vi "target.vi"() -> ()   [LabVIEW 2020]
uses:
  <vilib>/rvi/DataTransferAndStorage/Container/Common/niFpgaContainerGetUniqueNameForEmu.vi
  <vilib>/rvi/DataTransferAndStorage/Container/Common/niFpgaContainerSetEmuInfo.vi
  <vilib>/rvi/eio/common/nirviEmuReportErrorAndStop.vi
  <vilib>/rvi/Emulation/niFpgaGetClockAttributes.vi
  <vilib>/rvi/Emulation/niFpgaSctlEmulationGetInTimedLoop.vi
  <vilib>/rvi/Emulation/niFpgaEmulationReportErrorSimple.vi
  <vilib>/rvi/DataTransferAndStorage/Container/Common/niFpgaContainerExecOnDevCompGetState.vi
  <vilib>/rvi/Emulation/niFpgaEmulationIsFPGAContextNoSignature.vi
  <vilib>/rvi/errors/niFpgaSetErrorForExecOnDevCompSimple.vi
  <vilib>/rvi/FIFO/Fifo_Resource/nirvififoEmulationSetSize.vi
  <vilib>/rvi/FIFO/Fifo_Resource/nirviFifoEmulationQueueMgr.vi
  <instcachedir>/0/nirviFifoEmulationQueueMgr_E5CAEC123FF24DC58D834DCA3CDAA9B5.lvgen/nirviFifoEmulationQueueMgr_E5CAEC123FF24DC58D834DCA3CDAA9B5_004.vi
  <vilib>/rvi/FIFO/Fifo_Resource/nirvififoEmulationDetermineInputValidOut.vi
  <vilib>/rvi/FIFO/Fifo_Resource/nirvififoEmulationCreateLock.vi
  <vilib>/rvi/Emulation/niFpgaProcessEmulError.vi
  <vilib>/rvi/FIFO/Fifo_Resource/nirvififoEmulationObtainLock.vi
  <vilib>/rvi/FIFO/Fifo_Resource/nirvififoEmulationReleaseLock.vi
  <vilib>/rvi/occurrence/nirviWaitOnOccurrenceBase.vi
  <vilib>/rvi/errors/nirviReportUnexpectedCaseInternalError.vi
  <vilib>/rvi/errors/nirviReportUnexpectedCaseInternalError (U32).vi
  <vilib>/Utility/error.llb/Clear Errors.vi
  <vilib>/rvi/interface/RandomDataEmulation/niFpgaRandomDataHandleErrors.vi
  <vilib>/rvi/Emulation/niFpgaCriticalErrorInLSC.vi
  <vilib>/rvi/LocalResourceManager/LocalResourceManager.xnode
  <vilib>/rvi/DataTransferAndStorage/Container/XNode/niFpgaContainer.xnode
  <vilib>/rvi/FIFO/Fifo_Resource/niFpgaFifoEmulationRefIn.vi
  <vilib>/rvi/interface/RandomDataEmulation/nirviRandomDataFpgaReadWriteTemplate.vi
  <vilib>/eio/EIONode/EIONode.xnode
  <vilib>/rvi/eio/common/nirviEmuTemplateMethod_errors.vi
panel:
  out "x > y?":bool
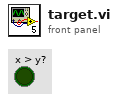
[diagram p1: front panel]
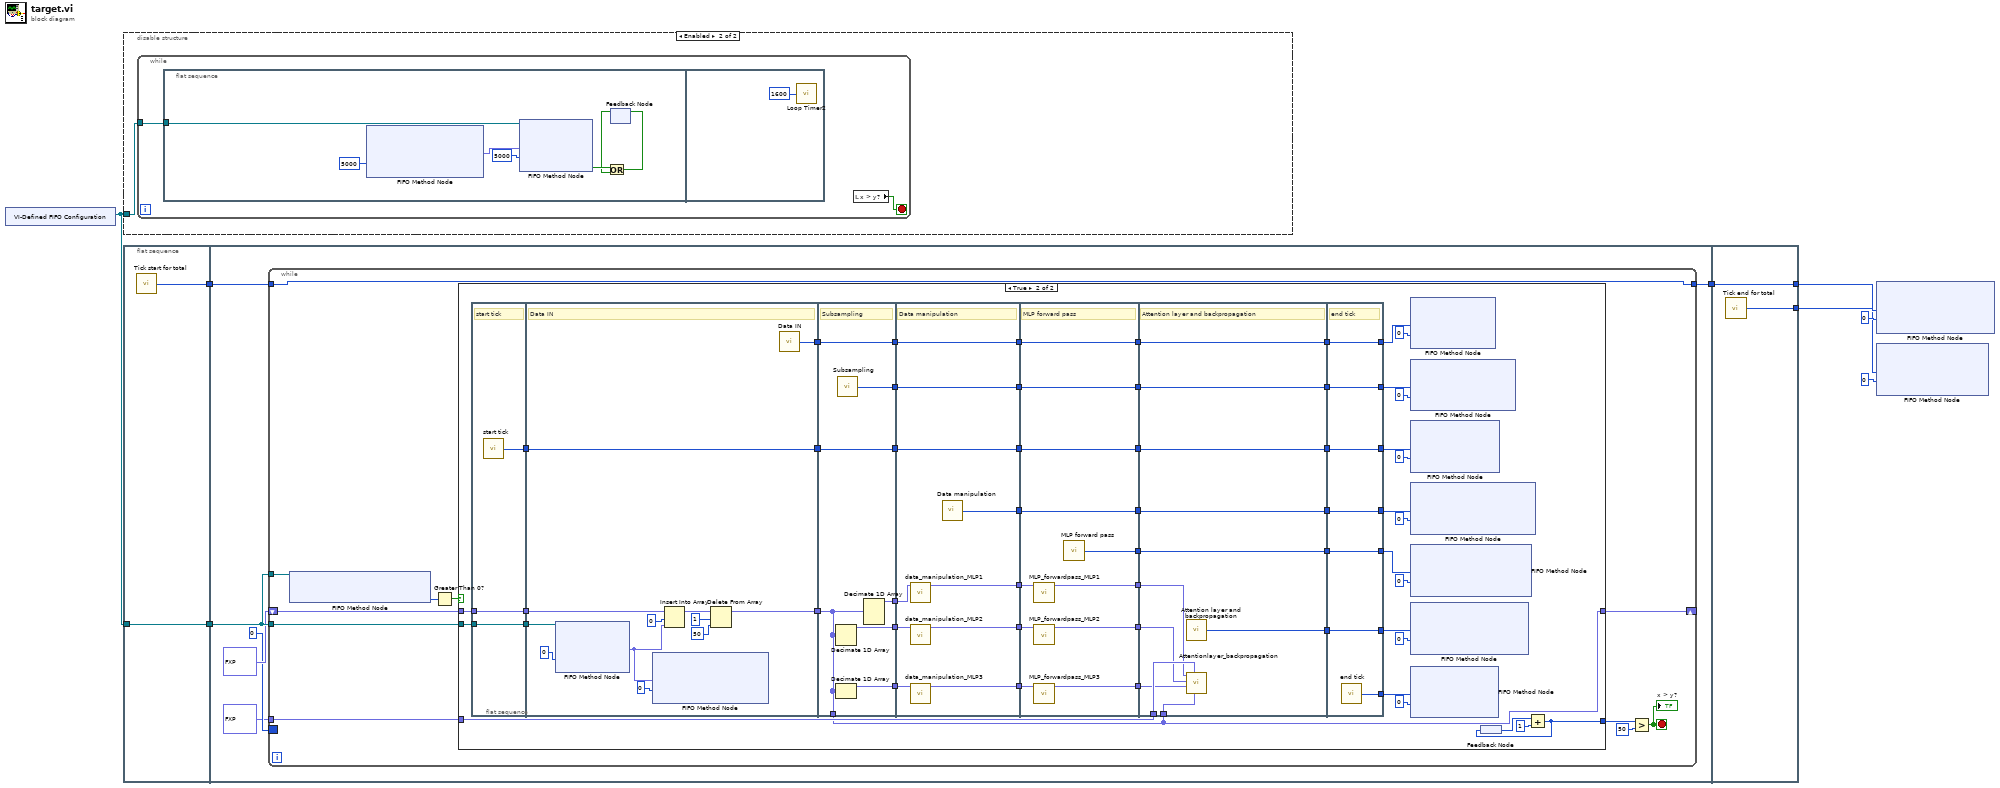
[diagram p0: block diagram]
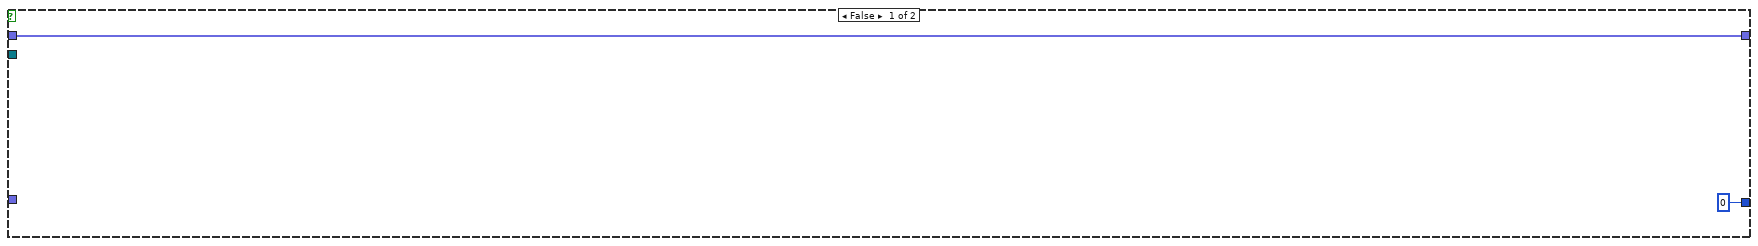
[diagram p2: hidden frame]
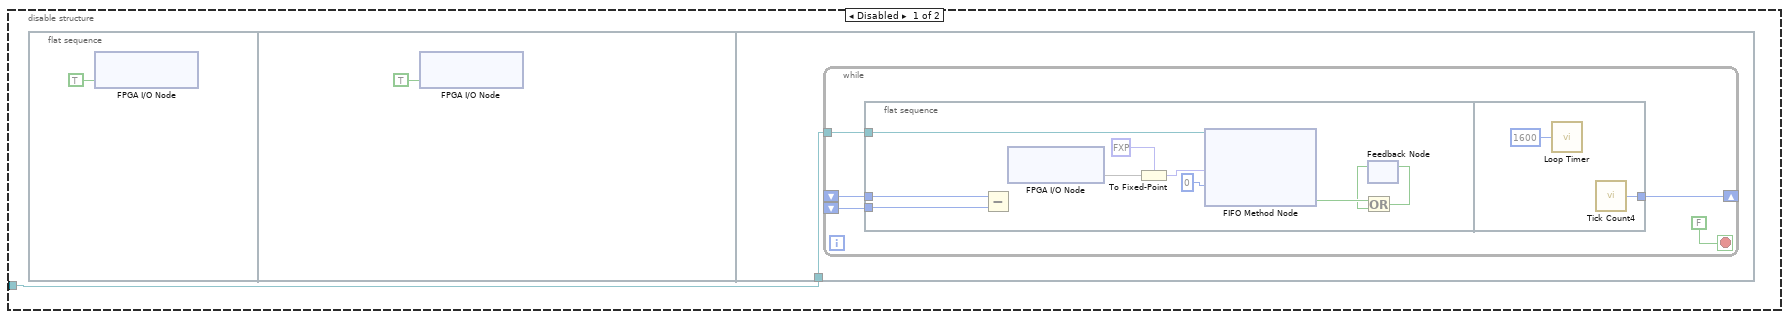
[diagram p3: hidden frame]
diagram:
  n1 = xnode "VI-Defined FIFO Configuration"() -> ("FIFO Out"=w8:refnum<k21>)
  n2 = disable-structure shown="Enabled" {
    disable-tunnel: w8 -> [w9 w30]
    frame Disabled {
      n3 = flat-sequence {
        tunnel: w9 -> [w12]
        frame #0 {
          n4 = xnode "FPGA I/O Node"("Mod1/Stop"=TRUE) -> ()  [unwired: 1 in, 1 out]
        }
        frame #1 {
          n5 = xnode "FPGA I/O Node"("Mod1/Start"=TRUE) -> ()  [unwired: 1 in, 1 out]
        }
        frame #2 {
          n6 = while {
            shift-right: [w17] -> _
            shift-left: _ -> [w16]
            shift-left: _ -> [w15]
            tunnel: w12 -> [w13]
            stop <- FALSE stop-if-true
            n7 = flat-sequence {
              tunnel: w16 -> [w27]
              tunnel: w15 -> [w26]
              tunnel: w13 -> [w18]
              tunnel: [w29] -> w17
              frame #0 {
                n8 = Subtract(x=w27, y=w26) -> ()  [unwired: 1 out]
                n9 = xnode "FPGA I/O Node"() -> ("Mod1/AI0"=w20)  [unwired: 1 in, 1 out]
                n10 = To Fixed-Point(fixed-point type=fxp<+/-,32,16> 0.0 ("f"), number=w20) -> (fixed-point=w19:fxp<+/-,32,16>)
                n11 = xnode ("FIFO Method Node")("Element"=w19, "Timeout"=0, "FIFO In"=w18) -> ("Timed Out?"=w24:bool)  [unwired: 1 in, 2 out]
                n12 = feedback #1() -> (w23:bool)  [unwired: 1 in]
                n13 = Or(x=w24, y=w23) -> (x .or. y?=w22:bool)
                n14 = feedback-in #1(w22) -> ()
              }
              frame #1 {
                n15 = call "Loop Timer"("Count(Ticks)"=u32 1600 ("Rate (uSec)")) -> ()  [unwired: 1 out]
                n16 = call "Tick Count4"() -> ("Tick Count(Ticks)"=w29:u32)
              }
            }
          }
        }
      }
    }
    frame Enabled {
      n17 = while {
        tunnel: w30 -> [w32]
        stop <- w31 stop-if-true
        n18 = flat-sequence {
          tunnel: w32 -> [w35]
          frame #0 {
            n19 = xnode ("FIFO Method Node")("Timeout"=5000) -> ("Element"=w33:fxp<+/-,32,16>)  [unwired: 1 in, 2 out]
            n20 = xnode ("FIFO Method Node")("Element"=w33, "Timeout"=5000, "FIFO In"=w35) -> ("Timed Out?"=w38:bool)  [unwired: 1 in, 2 out]
            n21 = feedback #2() -> (w37:bool)  [unwired: 1 in]
            n22 = Or(x=w38, y=w37) -> (x .or. y?=w36:bool)
            n23 = feedback-in #2(w36) -> ()
          }
          frame #1 {
            n24 = call "Loop Timer2"("Count(Ticks)"=u32 1600 ("Rate (uSec)")) -> ()  [unwired: 1 out]
          }
        }
        n25 = local read "x > y?"() -> (w31:bool)
      }
    }
  }
  n26 = flat-sequence {
    tunnel: w8 -> [w42]
    tunnel: [w42] -> w7
    tunnel: [w41] -> w3
    tunnel: w7 -> [w48]
    tunnel: w3 -> [w44]
    tunnel: [w43] -> w2
    tunnel: [w178] -> w5
    tunnel: w2 -> [w177]
    tunnel: [w177] -> w1
    frame #0 {
      n27 = call "Tick start for total"() -> ("Tick Count(Ticks)"=w41:u32)
    }
    frame #1 {
      n28 = while {
        tunnel: w48 -> [w58]
        tunnel: w48 -> [w55]
        border: 0 -> [_]
        shift-right: [w51] -> _
        shift-left: fxp<+/-,32,16>[] [0.0, 0.0, 0.0, 0.0, 0.0, 0.0, 0.0, 0.0, 0.0, 0.0, 0.0, 0.0, 0.0, 0.0, 0.0, 0.0, 0.0, 0.0, 0.0, 0.0, 0.0, 0.0, 0.0, 0.0, 0.0, 0.0, 0.0, 0.0, 0.0, 0.0, 0.0, 0.0, 0.0, 0.0, 0.0, 0.0, 0.0, 0.0, 0.0, 0.0, 0.0, 0.0, 0.0, 0.0, 0.0, 0.0, 0.0, 0.0, 0.0, 0.0] -> [w52]
        tunnel: fxp<+/-,32,16>[] [0.0, 0.0, 0.0, 0.0, 0.0, 0.0, 0.0, 0.0, 0.0, 0.0, 0.0, 0.0, 0.0, 0.0, 0.0, 0.0, 0.0, 0.0, 0.0, 0.0, 0.0, 0.0, 0.0, 0.0, 0.0] -> [w50]
        tunnel: w44 -> [w49]
        tunnel: [w49] -> w43
        stop <- w53 stop-if-true
        n29 = xnode ("FIFO Method Node")("FIFO In"=w58) -> ("Number of Elements to Read"=w59:u32)  [unwired: 1 in, 2 out]
        n30 = Greater Than 0?(x=w59) -> (x > 0?=w56:bool)
        n31 = case shown="True" w56 {
          tunnel: w55 -> [_ w115]
          tunnel: [0 w112] -> w54
          tunnel: w52 -> [w60 w111]
          tunnel: [w60 w85] -> w51
          tunnel: w50 -> [_ w98]
          frame False {
          }
          frame True {
            n32 = flat-sequence {
              tunnel: w111 -> [w117]
              tunnel: w115 -> [w118]
              tunnel: [w118] -> w110
              tunnel: [w117] -> w109
              tunnel: [w116] -> w65
              tunnel: w110 -> [w130]
              tunnel: w109 -> [w122]
              tunnel: [w121] -> w108
              tunnel: [w120] -> w71
              tunnel: [w119] -> w66
              tunnel: w65 -> [w119]
              tunnel: [w137] -> w85
              tunnel: w108 -> [w137]
              tunnel: [w136] -> w107
              tunnel: [w135] -> w106
              tunnel: [w134] -> w105
              tunnel: [w133] -> w76
              tunnel: w71 -> [w132]
              tunnel: [w132] -> w70
              tunnel: [w131] -> w67
              tunnel: w66 -> [w131]
              tunnel: w107 -> [w145]
              tunnel: w106 -> [w146]
              tunnel: w105 -> [w147]
              tunnel: [w144] -> w104
              tunnel: [w143] -> w103
              tunnel: [w142] -> w102
              tunnel: [w141] -> w81
              tunnel: [w140] -> w77
              tunnel: w76 -> [w140]
              tunnel: w70 -> [w139]
              tunnel: [w139] -> w69
              tunnel: [w138] -> w68
              tunnel: w67 -> [w138]
              tunnel: w104 -> [w158]
              tunnel: w103 -> [w157]
              tunnel: w102 -> [w156]
              tunnel: [w155] -> w101
              tunnel: [w154] -> w100
              tunnel: [w153] -> w99
              tunnel: [w152] -> w87
              tunnel: [w151] -> w84
              tunnel: w81 -> [w151]
              tunnel: [w150] -> w78
              tunnel: w77 -> [w150]
              tunnel: [w149] -> w72
              tunnel: w69 -> [w149]
              tunnel: w68 -> [w148]
              tunnel: [w148] -> w64
              tunnel: w101 -> [w165]
              tunnel: w100 -> [w166]
              tunnel: w99 -> [w167]
              tunnel: w98 -> [w169]
              tunnel: w85 -> [w168]
              tunnel: [w164] -> w90
              tunnel: w87 -> [w163]
              tunnel: [w163] -> w86
              tunnel: w84 -> [w162]
              tunnel: [w162] -> w83
              tunnel: [w161] -> w80
              tunnel: w78 -> [w161]
              tunnel: [w160] -> w74
              tunnel: w72 -> [w160]
              tunnel: w64 -> [w159]
              tunnel: [w159] -> w63
              tunnel: [w176] -> w91
              tunnel: w90 -> [w175]
              tunnel: [w175] -> w89
              tunnel: [w174] -> w88
              tunnel: w86 -> [w174]
              tunnel: w83 -> [w173]
              tunnel: [w173] -> w82
              tunnel: w80 -> [w172]
              tunnel: [w172] -> w79
              tunnel: w74 -> [w171]
              tunnel: [w171] -> w73
              tunnel: w63 -> [w170]
              tunnel: [w170] -> w62
              frame #0 {
                # "start tick"
                n33 = call "start tick"() -> ("Tick Count(Ticks)"=w116:u32)
              }
              frame #1 {
                # "Data IN"
                n34 = xnode ("FIFO Method Node")("Timeout"=0, "FIFO In"=w130) -> ("Element"=w123:fxp<+/-,32,16>)  [unwired: 1 in, 3 out]
                n35 = xnode ("FIFO Method Node")("Element"=w123, "Timeout"=0) -> ()  [unwired: 1 in, 2 out]
                n36 = Insert Into Array(array=w122, index=0, new element=w123) -> (w124:fxp<+/-,32,16>[])
                n37 = Delete From Array(array=w124, length=1, index=50) -> (array with subset deleted=w121:fxp<+/-,32,16>[])  [unwired: 1 out]
                n38 = call "Data IN"() -> ("Tick Count(Ticks)"=w120:u32)
              }
              frame #2 {
                # "Subsampling"
                n39 = Decimate 1D Array(w137) -> (w135:fxp<+/-,32,16>[])  [unwired: 3 out]
                n40 = Decimate 1D Array(w137) -> (w134:fxp<+/-,32,16>[])  [unwired: 2 out]
                n41 = call "Subsampling"() -> ("Tick Count(Ticks)"=w133:u32)
                n42 = Decimate 1D Array(w137) -> (w136:fxp<+/-,32,16>[])  [unwired: 4 out]
              }
              frame #3 {
                # "Data manipulation"
                n43 = call "data_manipulation_MLP1.vi"("Array in"=w145) -> ("Array out"=w142:fxp<+/-,64,35>[])  [unwired: 10 in]
                n44 = call "data_manipulation_MLP2.vi"("Array in"=w146) -> ("Array out"=w143:fxp<+/-,64,35>[])  [unwired: 10 in]
                n45 = call "data_manipulation_MLP3.vi"("Array in"=w147) -> ("Array out"=w144:fxp<+/-,64,35>[])  [unwired: 10 in]
                n46 = call "Data manipulation"() -> ("Tick Count(Ticks)"=w141:u32)
              }
              frame #4 {
                # "MLP forward pass"
                n47 = call "MLP_forwardpass_MLP1.vi"("Array in"=w156) -> ("Numeric"=w153:fxp<+/-,32,16>)  [unwired: 10 in]
                n48 = call "MLP_forwardpass_MLP2.vi"("Array in"=w157) -> ("Numeric"=w154:fxp<+/-,32,16>)  [unwired: 10 in]
                n49 = call "MLP_forwardpass_MLP3.vi"("Array in"=w158) -> ("Numeric"=w155:fxp<+/-,32,16>)  [unwired: 10 in]
                n50 = call "MLP forward pass"() -> ("Tick Count(Ticks)"=w152:u32)
              }
              frame #5 {
                # "Attention layer and backpropagation"
                n51 = call "Attention layer and backpropagation"() -> ("Tick Count(Ticks)"=w164:u32)
                n52 = call "Attentionlayer_backpropagation.vi"("Array"=w168, "Array 2"=w169, "Numeric"=w165, "Numeric 2"=w166, "Numeric 3"=w167) -> ()  [unwired: 7 in]
              }
              frame #6 {
                # "end tick"
                n53 = call "end tick"() -> ("Tick Count(Ticks)"=w176:u32)
              }
            }
            n54 = xnode ("FIFO Method Node")("Element"=w73, "Timeout"=0) -> ()  [unwired: 1 in, 2 out]
            n55 = xnode ("FIFO Method Node")("Element"=w79, "Timeout"=0) -> ()  [unwired: 1 in, 2 out]
            n56 = xnode ("FIFO Method Node")("Element"=w62, "Timeout"=0) -> ()  [unwired: 1 in, 2 out]
            n57 = xnode ("FIFO Method Node")("Element"=w82, "Timeout"=0) -> ()  [unwired: 1 in, 2 out]
            n58 = xnode ("FIFO Method Node")("Element"=w88, "Timeout"=0) -> ()  [unwired: 1 in, 2 out]
            n59 = xnode ("FIFO Method Node")("Element"=w89, "Timeout"=0) -> ()  [unwired: 1 in, 2 out]
            n60 = xnode ("FIFO Method Node")("Element"=w91, "Timeout"=0) -> ()  [unwired: 1 in, 2 out]
            n61 = feedback #3() -> (w113:i32)
            n62 = Add(x=w113, y=1) -> (x+y=w112:i32)
            n63 = feedback-in #3(w112) -> ()
          }
        }
        n64 = Greater?(x=w54, y=50) -> (0:w53:bool)
        "x > y?" <- w53
      }
    }
    frame #2 {
      n65 = call "Tick end for total"() -> ("Tick Count(Ticks)"=w178:u32)
    }
  }
  n66 = xnode ("FIFO Method Node")("Element"=w5, "Timeout"=0) -> ()  [unwired: 1 in, 2 out]
  n67 = xnode ("FIFO Method Node")("Element"=w1, "Timeout"=0) -> ()  [unwired: 1 in, 2 out]
